vi "mecanum_tank_1.vi"   [LabVIEW 2012, in "Mecanum Drive.lvrbt"]
uses:
  Mecanum Drive.lvrbt
  <vilib>/NXT/Hardware/Plugins/Tetrix 180 deg Servo/Tetrix180ServoAddress.ctl
  <vilib>/NXT/Hardware/Plugins/Tetrix DC Motor/TetrixDCMotorAddress.ctl
  <vilib>/NXT/NXTIO Xnodes/NXTIONodeSubVIs/TETRIX IO Move Servos.vi
  <vilib>/NXT/NXTIO Xnodes/NXTIONodeSubVIs/TETRIX IO Move DC Motors.vi
  <vilib>/NXT/Dual Mode Library/Display/drawNumber.vi
  <vilib>/NXT/NXTIO Xnodes/NXTIONodeSubVIs/TETRIX IO Check Battery.vi
  <vilib>/NXT/NXTIO Xnodes/NXTIONodeSubVIs/TETRIX IO Stop DC Motors.vi
  <vilib>/NXT/NXTIO Xnodes/AddressXNode/NXTIOAddress.xnode
  <vilib>/NXT/Subs/LVHSConnector.ctl
  <vilib>/NXT/NXTIO Xnodes/NXTIOXNode/NXTIO.xnode
  <vilib>/NXT/LegoClasses/BrickReference/BrickReference.lvclass
panel:
  # "This VI was generated based on your configuration in the Remote Control Editor. You may modify the code as needed for your robot. To test this program for an FTC match, return to the Remote Control Editor, select the \"Run Program\" tab, and choose \"Teleop\"."
types:
  T1 = typedef "Tetrix180ServoAddress.ctl" = i32
  T2 = typedef "TetrixDCMotorAddress.ctl" = i32
  T3 = cluster{"TetrixDCMotor":T2, "TetrixDCMotor 2":T2}
  T4 = typedef "LVHSConnector.ctl" = refnum<class "BrickReference.lvclass">
  T5 = typedef "FTC ControllerState.ctl" = cluster{"Left X":i8, "Left Y":i8, "Right X":i8, "Right Y":i8, "Button Encoding 9-12":u8, "Button Encoding 1-8":u8, "POV":T6}
  T6 = typedef "FTC POVState.ctl" = i8
  T7 = typedef "FTC ButtonEventType.ctl" = enum16{"Pressed", "Released"}
  T8 = cluster{"Button ID":enum16{"None", "Button 1", "Button 2", "Button 3", "Button 4", "Button 5", "Button 6", "Button 7", "Button 8", "Button 9", "Button 10", "Button 11", "Button 12", "POV Up", "POV Up Right", "POV Right", "POV Down Right", "POV Down", "POV Down Left", "POV Left", "POV Up Left"}, "Event Type":T7}[]
  T9 = typedef "FTC ButtonState.ctl" = cluster{"Button 1":bool, "Button 2":bool, "Button 3":bool, "Button 4":bool, "Button 5":bool, "Button 6":bool, "Button 7":bool, "Button 8":bool, "Button 9":bool, "Button 10":bool, "Button 11":bool, "Button 12":bool, "POV":T6}
  T10 = enum16{"None", "Button 1", "Button 2", "Button 3", "Button 4", "Button 5", "Button 6", "Button 7", "Button 8", "Button 9", "Button 10", "Button 11", "Button 12", "POV Up", "POV Up Right", "POV Right", "POV Down Right", "POV Down", "POV Down Left", "POV Left", "POV Up Left"}
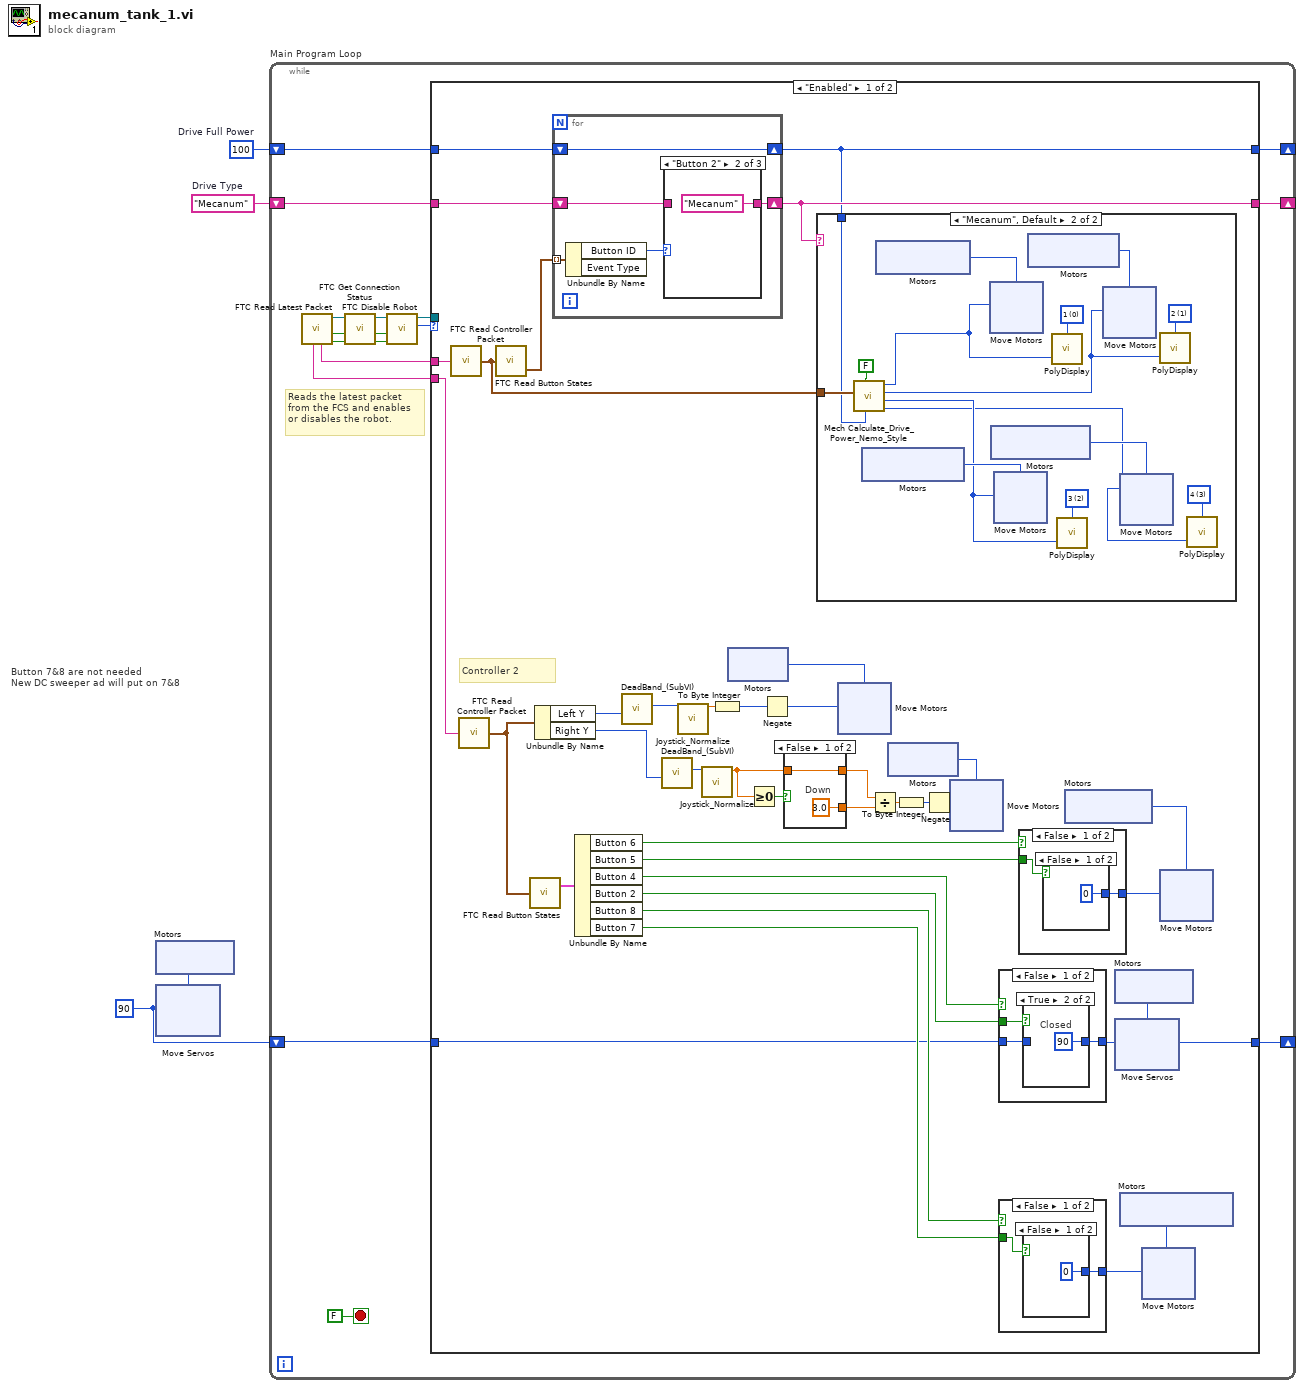
[diagram p0: block diagram]
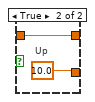
[diagram p2: hidden frame]
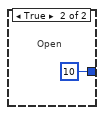
[diagram p4: hidden frame]
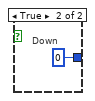
[diagram p5: hidden frame]
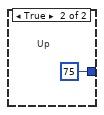
[diagram p6: hidden frame]
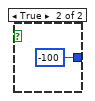
[diagram p7: hidden frame]
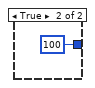
[diagram p8: hidden frame]
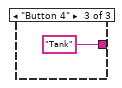
[diagram p11: hidden frame]
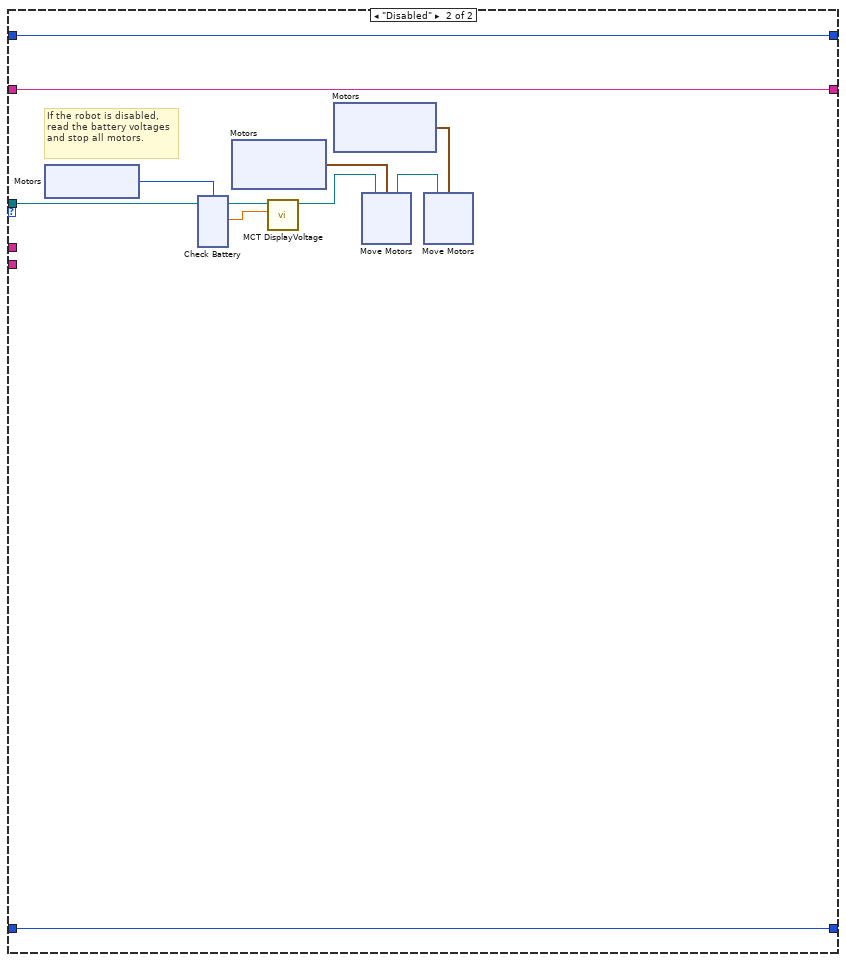
[diagram p12: hidden frame]
diagram:
  w1 = u8 90 ("Position 1")
  w3 = 100  # Drive Full Power
  w4 = "Mecanum"  # Drive Type
  # "Button 7&8 are not needed\nNew DC sweeper ad will put on 7&8"
  n1 = xnode "Motors"() -> ("Motor"=w2:T1)
  n2 = xnode "Move Servos"("Position 1"=w1, "Motors"=w2) -> ()  [unwired: 1 in, 1 out]
  n3 = while "Main Program Loop" {
    shift-right: [w9] -> _
    shift-left: w4 -> [w10]
    shift-right: [w7] -> _
    shift-left: w3 -> [w8]
    shift-right: [w5] -> _
    shift-left: w1 -> [w6]
    stop <- FALSE stop-if-true
    # "Reads the latest packet\nfrom the FCS and enables\nor disables the robot."
    n4 = call <vilib>:"FTC Read Latest Packet.vi"() -> ("Packet Received?"=w18:bool, "Stopped?"=w15:bool, "NXT"=w17:T4, "Controller 1"=w20:string, "Controller 2"=w19:string)  [unwired: 6 in, 1 out]
    n5 = call <vilib>:"FTC Get Connection Status.vi"("Packet Received?"=w18, "Stopped?"=w15, "NXT"=w17) -> ("Online?"=w12:bool, "Stopped?"=w13:bool, "NXT"=w14:T4)  [unwired: 5 in]
    n6 = call <vilib>:"FTC Disable Robot.vi"("Online?"=w12, "Stopped?"=w13, "NXT"=w14) -> ("Enabled?"=w16:enum16{"Disabled", "Enabled"}, "NXT"=w11:T4)  [unwired: 3 in]
    n7 = case "disableCase" shown="\"Enabled\"" w16 {
      tunnel: w20 -> [w60 _]
      tunnel: w19 -> [w59 _]
      tunnel: w11 -> [_ w186]
      tunnel: w10 -> [w57 w178]
      tunnel: [w56 w178] -> w9
      tunnel: w8 -> [w54 w177]
      tunnel: [w53 w177] -> w7
      tunnel: w6 -> [w31 w176]
      tunnel: [w34 w176] -> w5
      frame "Enabled" {
        # "Controller 2"
        n8 = call <vilib>:"FTC Read Controller Packet.vi"("Packet"=w60) -> ("Controller State"=w55:T5)  [unwired: 4 in]
        n9 = call <vilib>:"FTC Read Controller Packet.vi"("Packet"=w59) -> ("Controller State"=w46:T5)  [unwired: 4 in]
        n10 = call <vilib>:"FTC Read Button States.vi"("Controller State"=w55) -> ("Button Events"=w58:T8)  [unwired: 2 in, 1 out]
        n11 = call <vilib>:"FTC Read Button States.vi"("Controller State"=w46) -> ("Button States"=w45:T9)  [unwired: 2 in, 1 out]
        n12 = Unbundle By Name(w46) -> ("Left Y"=w52:i8, "Right Y"=w47:i8)
        n13 = for {
          tunnel: w58 -> [w172] mode=indexing
          shift-right: [w170] -> w56
          shift-left: w57 -> [w169]
          shift-right: [w168] -> w53
          shift-left: w54 -> [w168]
          n14 = Unbundle By Name(w172) -> ("Button ID"=w171:T10)  [unwired: 1 out]
          n15 = case shown="\"Button 2\"" w171 {
            tunnel: [w173 "Mecanum" "Tank"] -> w170
            tunnel: w169 -> [w173 _ _]
            frame "None", Default {
            }
            frame "Button 2" {
            }
            frame "Button 4" {
            }
          }
        }
        n16 = Unbundle By Name(w45) -> ("Button 6"=w42:bool, "Button 5"=w41:bool, "Button 4"=w32:bool, "Button 2"=w33:bool, "Button 8"=w37:bool, "Button 7"=w36:bool)
        n17 = call "DeadBand_(SubVI).vi"("Axis In"=w52) -> ("Axis out"=w51:i8)  [unwired: 10 in]
        n18 = call "DeadBand_(SubVI).vi"("Axis In"=w47) -> ("Axis out"=w48:i8)  [unwired: 10 in]
        n19 = call "Joystick_Normalize.vi"("Joystick In"=w51) -> ("Norm Out"=w50:sgl)  [unwired: 10 in]
        n20 = call "Joystick_Normalize.vi"("Joystick In"=w48) -> ("Norm Out"=w25:sgl)  [unwired: 10 in]
        n21 = To Byte Integer(number=w50) -> (8bit integer=w28:i8)
        n22 = xnode "Motors"() -> ("Motor"=w49:T2)
        n23 = Greater Or Equal To 0?(x=w25) -> (x >= 0?=w26:bool)
        n24 = Negate(x=w28) -> (-x=w27:i8)
        n25 = case shown="False" w26 {
          tunnel: [w69 w71] -> w23
          tunnel: w25 -> [w69 w71]
          tunnel: [3.0 10.0] -> w24
          frame False {
            # "Down"
          }
          frame True {
            # "Up"
          }
        }
        n26 = case shown="\"Mecanum\", Default" w56 {
          tunnel: w55 -> [_ w123]
          tunnel: w53 -> [_ w121]
          frame "Tank" {
          }
          frame "Mecanum", Default {
            w125 = i16 3 items=["1", "2", "3", "4", "5", "6", "7", "8", "9", "10", "11", "12"] ("Line")
            w127 = i16 2 items=["1", "2", "3", "4", "5", "6", "7", "8", "9", "10", "11", "12"] ("Line")
            w129 = i16 1 items=["1", "2", "3", "4", "5", "6", "7", "8", "9", "10", "11", "12"] ("Line")
            w130 = i16 0 items=["1", "2", "3", "4", "5", "6", "7", "8", "9", "10", "11", "12"] ("Line")
            n27 = call "Mech Calculate_Drive_Power_Nemo_Style.vi"("Power"=w121, "Reverse"=FALSE, "Controller State"=w123) -> ("Right Rear Power"=w124:i8, "Right Front Power"=w126:i8, "Left Rear Power"=w128:i8, "Left Front Power"=w122:i8)  [unwired: 5 in]
            n28 = xnode ("Motors")() -> ("Motor"=w135:T2)
            n29 = xnode ("Motors")() -> ("Motor"=w132:T2)
            n30 = xnode ("Move Motors")("Power/Speed 1"=w122, "Motors"=w132) -> ()  [unwired: 1 in, 1 out]
            n31 = xnode ("Motors")() -> ("Motor"=w134:T2)
            n32 = xnode ("Move Motors")("Power/Speed 1"=w126, "Motors"=w135) -> ()  [unwired: 1 in, 1 out]
            n33 = xnode ("Motors")() -> ("Motor"=w133:T2)
            n34 = call-poly <vilib>:"PolyDisplay.vi"("number"=w122, "Line"=w130) -> ()  [unwired: 2 in, 1 out]
            n35 = call-poly <vilib>:"PolyDisplay.vi"("number"=w126, "Line"=w127) -> ()  [unwired: 2 in, 1 out]
            n36 = xnode ("Move Motors")("Power/Speed 1"=w128, "Motors"=w133) -> ()  [unwired: 1 in, 1 out]
            n37 = xnode ("Move Motors")("Power/Speed 1"=w124, "Motors"=w134) -> ()  [unwired: 1 in, 1 out]
            n38 = call-poly <vilib>:"PolyDisplay.vi"("number"=w128, "Line"=w129) -> ()  [unwired: 2 in, 1 out]
            n39 = call-poly <vilib>:"PolyDisplay.vi"("number"=w124, "Line"=w125) -> ()  [unwired: 2 in, 1 out]
          }
        }
        n40 = xnode "Move Motors"("Power/Speed 1"=w27, "Motors"=w49) -> ()  [unwired: 1 in, 1 out]
        n41 = Divide(x=w23, y=w24) -> (x/y=w29:dbl)
        n42 = xnode "Motors"() -> ("Motor"=w44:T2)
        n43 = To Byte Integer(number=w29) -> (8bit integer=w43:i8)
        n44 = Negate(x=w43) -> (-x=w30:i8)
        n45 = xnode "Move Motors"("Power/Speed 1"=w30, "Motors"=w44) -> ()  [unwired: 1 in, 1 out]
        n46 = case shown="False" w32 {
          tunnel: w33 -> [w74 _]
          tunnel: [w73 u8 10] -> w34
          tunnel: w31 -> [w72 _]
          frame False {
            n47 = case shown="True" w74 {
              tunnel: [w75 u8 90] -> w73
              tunnel: w72 -> [w75 _]
              frame False {
              }
              frame True {
                # "Closed"
              }
            }
          }
          frame True {
            # "Open"
          }
        }
        n48 = case shown="False" w37 {
          tunnel: w36 -> [w87 _]
          tunnel: [w86 u8 75] -> w22
          frame False {
            n49 = case shown="False" w87 {
              tunnel: [u8 0 u8 0] -> w86
              frame False {
              }
              frame True {
                # "Down"
              }
            }
          }
          frame True {
            # "Up"
          }
        }
        n50 = case shown="False" w42 {
          tunnel: w41 -> [w101 _]
          tunnel: [w100 i8 100] -> w39
          frame False {
            n51 = case shown="False" w101 {
              tunnel: [i8 0 i8 -100] -> w100
              frame False {
              }
              frame True {
              }
            }
          }
          frame True {
          }
        }
        n52 = xnode "Motors"() -> ("Motor"=w40:T2)
        n53 = xnode "Motors"() -> ("Motor"=w35:T1)
        n54 = xnode "Move Servos"("Position 1"=w34, "Motors"=w35) -> ()  [unwired: 1 in, 1 out]
        n55 = xnode "Motors"() -> ("Motor"=w38:T2)
        n56 = xnode "Move Motors"("Power/Speed 1"=w22, "Motors"=w38) -> ()  [unwired: 1 in, 1 out]
        n57 = xnode "Move Motors"("Power/Speed 1"=w39, "Motors"=w40) -> ()  [unwired: 1 in, 1 out]
      }
      frame "Disabled" {
        # "If the robot is disabled, read the battery voltages and stop all motors."
        n58 = xnode ("Motors")() -> ("Motor"=w185:T2)
        n59 = xnode ("Check Battery")("Motors"=w185, "NXT/EV3"=w186) -> ("Voltage 1"=w184:sgl, "NXT/EV3"=w183:T4)
        n60 = xnode "Motors"() -> ("Motor"=w182:cluster{"TetrixDCMotor":T2, "TetrixDCMotor":T2})
        n61 = call <vilib>:"MCT DisplayVoltage.vi"("Motor Voltage"=w184, "NXT"=w183) -> ("NXT"=w181:T4)  [unwired: 9 in]
        n62 = xnode "Motors"() -> ("Motor"=w180:cluster{"TetrixDCMotor":T2, "TetrixDCMotor":T2})
        n63 = xnode "Move Motors"("Motors"=w182, "NXT/EV3"=w181) -> ("NXT/EV3"=w179:T4)
        n64 = xnode "Move Motors"("Motors"=w180, "NXT/EV3"=w179) -> ()  [unwired: 1 out]
      }
    }
  }
